vi "Signal Generation stage scanning.vi"(1 "Laser 2 Amplitude":dbl=2.0 caption="Amplitude 2" format="%0.2p", 3 "Acquisition type":T1(ring), 4 "Laser 1 duration":dbl caption="Desired Duration" format="%.2f", 5 "Laser 2 duration":dbl caption="Desired Duration" format="%.2f", 6 "Laser 1 Amplitude":dbl=2.0 caption="Amplitude" format="%0.2p", 7 "Resulting sample clock rate":dbl, 10 "Camera 1 Delay (ms)":dbl, 12 "Laser 2 Delay":dbl) -> (11 "DO task":u32[][](array[numeric]), 13 "Total samples":dbl format="%.2f", 16 "AO task":dbl[][](array[numeric]))   [LabVIEW 2020]
doc: "This subVI is used to create a Sine, Square, Triangle or Sawtooth Waveform. The inputs to this VI are the Waveform Type, which determines if the output waveform is a Sine, Square, Triangle, or Sawtooth Waveform, the amplitude, Desired Frequency, Samples per Buffer, and Cycles per Buffer. \n\nThe Desired Frequency, Samples per Buffer, and Cycles per Buffer are used to calculate the sample clock rate. The DAQmx Timing property node sets the sample clock rate for the device specified in the task/channels in control. \n\nThe actual, coerced, sample clock rate is returned and used as an input to the Basic Function Generator.vi. The Basic Function Generator returns a waveform of data with timing information.\n\nThe formula below was used to determine the sample clock rate:\n\nDesired Frequency=[(Cycles/Buffer)X(Sample Clock Rate)]/Samples per Buffer\n\nNote: The Block Diagram rearranges the variables to solve for Sample Clock Rate"
panel:
  out "output array":dbl[][](array[numeric])
  out "initialized array":dbl[][](array[numeric])
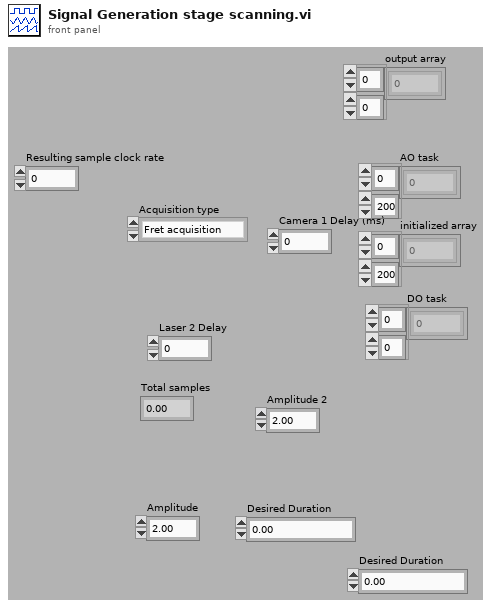
[diagram p1: front panel]
types:
  T1 = enum16{"Fret acquisition", "Alternate acquisition", "Simultaneous acquisition"}
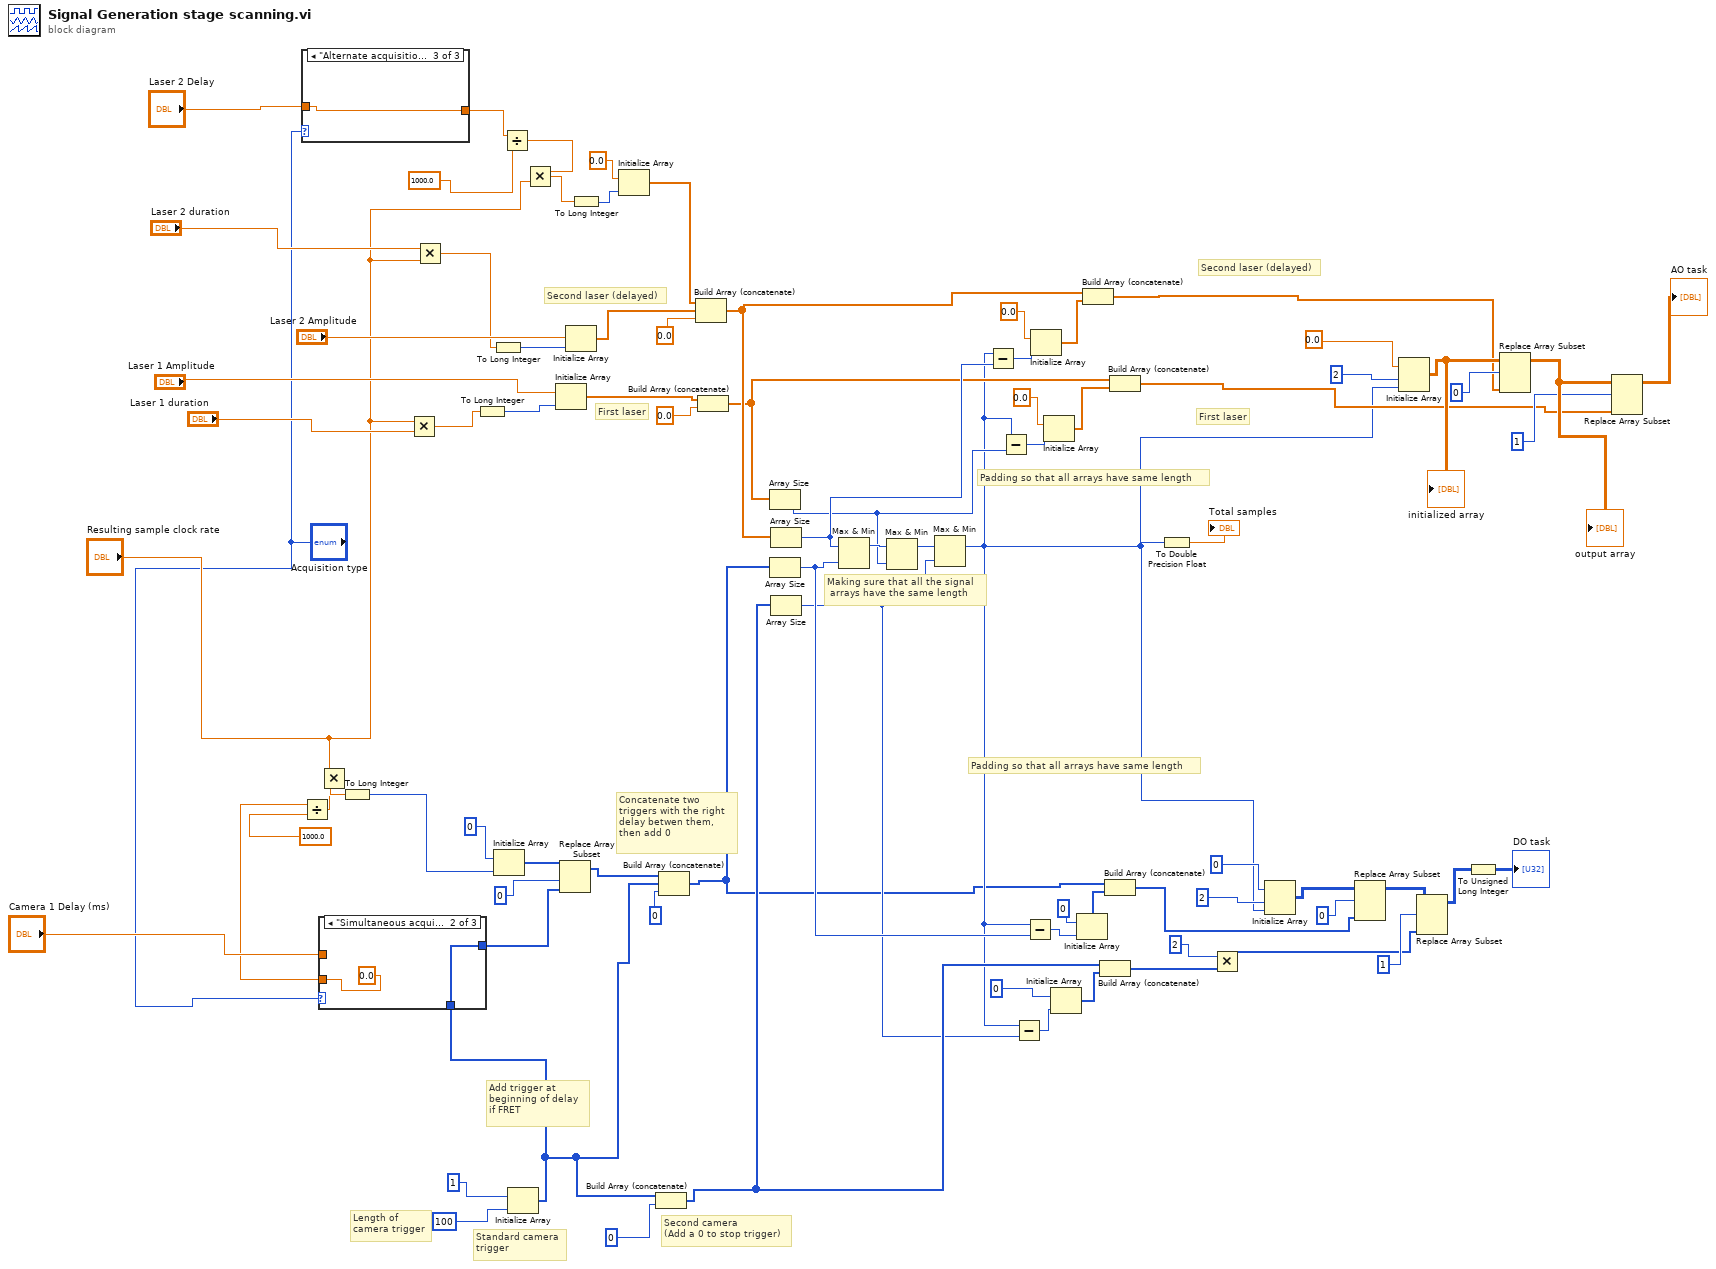
[diagram p0: block diagram]
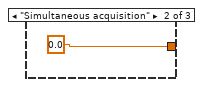
[diagram p3: hidden frame]
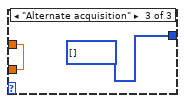
[diagram p5: hidden frame]
diagram:
  # "Add trigger at \nbeginning of delay\nif FRET"
  # "Second camera\n(Add a 0 to stop trigger)"
  # "Length of \ncamera trigger"
  # "Standard camera\ntrigger"
  # "Concatenate two \ntriggers with the right \ndelay betwen them, \nthen add 0"
  # "Second laser (delayed)"
  # "First laser"
  # "Padding so that all arrays have same length"
  # "Padding so that all arrays have same length"
  # "Making sure that all the signal\n arrays have the same length"
  # "Second laser (delayed)"
  # "First laser"
  n1 = case shown="\"Alternate acquisition\"" "Acquisition type" {
    tunnel: "Laser 2 Delay" -> [w84 _ w86]
    tunnel: [w84 0.0 ("y") w86] -> w2
    frame "Fret acquisition", Default {
    }
    frame "Simultaneous acquisition" {
    }
    frame "Alternate acquisition" {
    }
  }
  n2 = Multiply(x="Resulting sample clock rate", y="Laser 1 duration") -> (x*y=w81:dbl)
  n3 = Multiply(x="Laser 2 duration", y="Resulting sample clock rate") -> (x*y=w10:dbl)
  n4 = To Long Integer(number=w81) -> (32bit integer=w16:i32)
  n5 = To Long Integer(number=w10) -> (32bit integer=w13:i32)
  n6 = Divide(x=w2, y=1000.0) -> (x/y=w78:dbl)
  n7 = Initialize Array(1 ("new element/subarray"), 100 ("dimension size")) -> (w8:i32[])
  n8 = case shown="\"Simultaneous acquisition\"" "Acquisition type" {
    tunnel: w8 -> [w88 w90 _]
    tunnel: [w88 w90 i32[] []] -> w6
    tunnel: "Camera 1 Delay (ms)" -> [w87 _ w91]
    tunnel: [w87 0.0 ("y") w91] -> w4
    frame "Fret acquisition", Default {
    }
    frame "Simultaneous acquisition" {
    }
    frame "Alternate acquisition" {
    }
  }
  n9 = Divide(x=w4, y=1000.0) -> (x/y=w72:dbl)
  n10 = Multiply(x="Resulting sample clock rate", y=w72) -> (x*y=w74:dbl)
  n11 = To Long Integer(number=w74) -> (32bit integer=w7:i32)
  n12 = Initialize Array(0, w7) -> (w43:i32[])
  n13 = Multiply(x=w78, y="Resulting sample clock rate") -> (x*y=w75:dbl)
  n14 = Initialize Array("Laser 1 Amplitude", w16) -> (w54:dbl[])
  n15 = Replace Array Subset(array=w43, new element=w6, index=0) -> (w41:i32[])
  n16 = Initialize Array("Laser 2 Amplitude", w13) -> (w14:dbl[])
  n17 = To Long Integer(number=w75) -> (32bit integer=w76:i32)
  n18 = Initialize Array(0.0 ("element"), w76) -> (w80:dbl[])
  n19 = Build Array (concatenate)(w8, 0) -> (w46:i32[])
  n20 = Build Array (concatenate)(w41, w8, 0) -> (w9:i32[])
  n21 = Build Array (concatenate)(w80, w14, 0.0) -> (w67:dbl[])
  n22 = Build Array (concatenate)(w54, 0.0) -> (w50:dbl[])
  n23 = Array Size(array=w50) -> (size(s)=w47:i32)
  n24 = Array Size(array=w9) -> (size(s)=w63:i32)
  n25 = Array Size(array=w67) -> (size(s)=w66:i32)
  n26 = Array Size(array=w46) -> (size(s)=w45:i32)
  n27 = Max & Min(x=w66, y=w63) -> (max(x,y)=w48:i32)  [unwired: 1 out]
  n28 = Max & Min(x=w48, y=w47) -> (max(x,y)=w49:i32)  [unwired: 1 out]
  n29 = Max & Min(x=w49, y=w45) -> (max(x,y)=w24:i32)  [unwired: 1 out]
  n30 = Subtract(x=w24, y=w66) -> (x-y=w68:i32)
  n31 = Subtract(x=w24, y=w47) -> (x-y=w53:i32)
  n32 = Subtract(x=w24, y=w45) -> (x-y=w64:i32)
  n33 = Subtract(x=w24, y=w63) -> (x-y=w70:i32)
  n34 = Initialize Array(0.0, w68) -> (w69:dbl[])
  n35 = Initialize Array(0.0, w53) -> (w51:dbl[])
  n36 = Initialize Array(0, w64) -> (w65:i32[])
  n37 = Initialize Array(0, w70) -> (w44:i32[])
  n38 = Build Array (concatenate)(w67, w69) -> (w26:dbl[])
  n39 = Build Array (concatenate)(w46, w65) -> (w18:i32[])
  n40 = Build Array (concatenate)(w9, w44) -> (w35:i32[])
  n41 = Build Array (concatenate)(w50, w51) -> (w25:dbl[])
  n42 = To Double Precision Float(number=w24) -> (double precision float=→"Total samples":dbl)
  n43 = Multiply(x=2 ("dimension size"), y=w18) -> (x*y=w19:i32[])
  n44 = Initialize Array(0 ("dimension size"), 2 ("dimension size"), w24) -> (w38:i32[][])
  n45 = Replace Array Subset(array=w38, new element=w35, index (row)=0 ("dimension size")) -> (w37:i32[][])  [unwired: 1 in]
  n46 = Initialize Array(0.0, 2 ("dimension size"), w24) -> (w30:dbl[][])
  "initialized array" <- w30
  n47 = Replace Array Subset(array=w37, new element=w19, index (row)=1 ("dimension size")) -> (w36:i32[][])  [unwired: 1 in]
  n48 = To Unsigned Long Integer(number=w36) -> (unsigned 32bit integer=→"DO task":u32[][])
  n49 = Replace Array Subset(array=w30, new element=w26, index (row)=0 ("dimension size")) -> (w29:dbl[][])  [unwired: 1 in]
  "output array" <- w29
  n50 = Replace Array Subset(array=w29, new element=w25, index (row)=1 ("dimension size")) -> (→"AO task":dbl[][])  [unwired: 1 in]
